vi "InitializeAnalogOutput.vi"(1 "AOTF":u16(ring) items=["None", "Laser 1", "Laser 2", "Laser 1 + 2", "Laser 3", "Laser 1 + 3", "Laser 2 + 3", "Laser 1+2+3", "Laser 1+2+3+4", "Laser 2+3+4"], 2 "% puls-duration":dbl=95.0, 3 "Image Settings":T1={"Start Position (µm)"={"x"=0.0, "y"=0.0, "z"=0.0}, "End Position (µm)"={"x"=10.0, "y"=10.0, "z"=0.0}, "Image Resolution (nm/pixel)"={"x"=50.0, "y"=50.0, "z"=100.0}, "Image Size (µm)"={"x"=10.0, "y"=10.0, "z"=0.0}, "Image Size (pixel)"={"x"=50, "y"=50, "z"=0}, "Time Resolution\n(ms/pixel)"=7.0, "1st Axis"=0, "2nd Axis"=1, "Retrace"=FALSE, "Estimated Time"=""} {"2nd Axis" items=["x", "y", "z"]; "1st Axis" items=["x", "y", "z"]; "Time Resolution\n(ms/pixel)" format="%.2f"; "Image Resolution (nm/pixel)"."z" format="%.2f"; "Image Resolution (nm/pixel)"."y" format="%.2f"; "Image Resolution (nm/pixel)"."x" format="%.2f"; "Image Size (µm)"."z" format="%.2f"; "Image Size (µm)"."y" format="%.2f"; "Image Size (µm)"."x" format="%.2f"; "End Position (µm)"."z" format="%.2f"; "End Position (µm)"."y" format="%.2f"; "End Position (µm)"."x" format="%.2f"; "Start Position (µm)"."z" format="%.2f"; "Start Position (µm)"."y" format="%.2f"; "Start Position (µm)"."x" format="%.2f"}, 4 "EOM":u16(ring) items=["None", "Trace", "Retrace", "All"]) -> (0 "Error out":errorcluster)   [LabVIEW 2009]
uses:
  ImageSettings.ctt
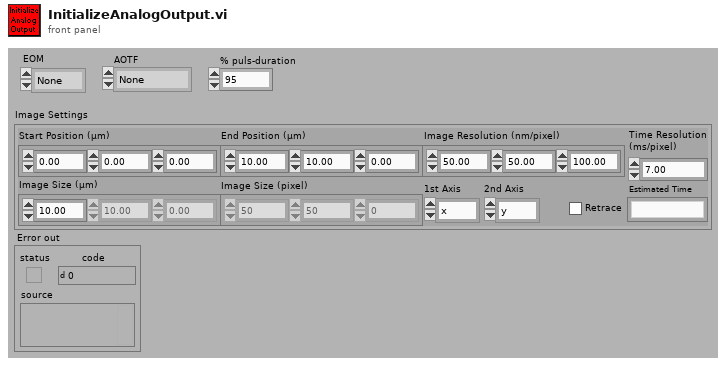
[diagram p1: front panel]
types:
  T1 = typedef "ImageSettings.ctt" = cluster{"Start Position (µm)":cluster{"x":dbl, "y":dbl, "z":dbl}, "End Position (µm)":cluster{"x":dbl, "y":dbl, "z":dbl}, "Image Resolution (nm/pixel)":cluster{"x":dbl, "y":dbl, "z":dbl}, "Image Size (µm)":cluster{"x":dbl, "y":dbl, "z":dbl}, "Image Size (pixel)":cluster{"x":u32, "y":u32, "z":u32}, "Time Resolution\n(ms/pixel)":dbl, "1st Axis":u16, "2nd Axis":u16, "Retrace":bool, "Estimated Time":string}
  T2 = typedef "AnalogSettings.ctt" = cluster{"PCI 671x Device Number":u32, "Samples per Unit":u32}
  T3 = typedef "AnalogTrace.ctt" = cluster{"Used":bool, "Waveform":waveform(dbl)}
  T4 = cluster{"new plane step[0]":dbl, "new plane step[1]":dbl, "new plane step[2]":dbl}
  T5 = typedef "LineScanStatus.ctt" = cluster{"in line":bool, "line status":cluster{"count":u32, "current":cluster{"x":u32, "y":u32, "z":u32}}, "plane status":cluster{"count":u32, "current":cluster{"x":u32, "y":u32, "z":u32}}, "new line step":cluster{"x":dbl, "y":dbl, "z":dbl}, "new plane step":cluster{"x":dbl, "y":dbl, "z":dbl}}
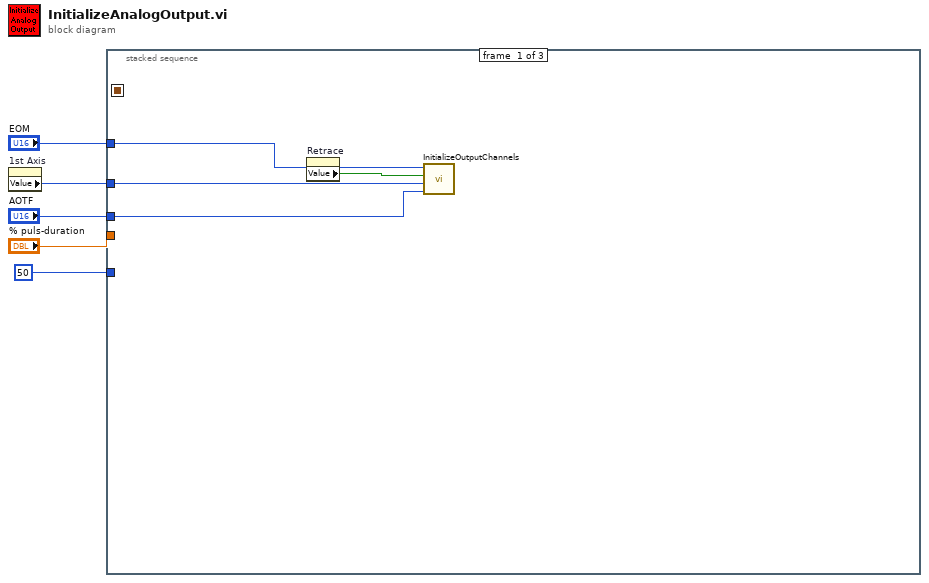
[diagram p0: block diagram]
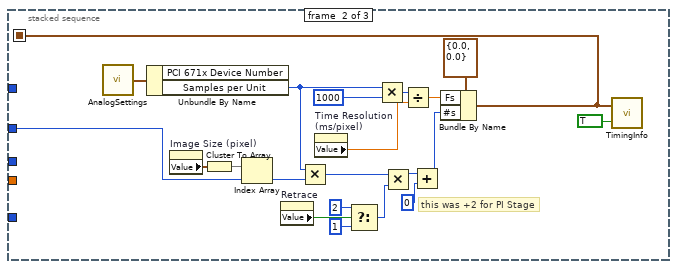
[diagram p2: hidden frame]
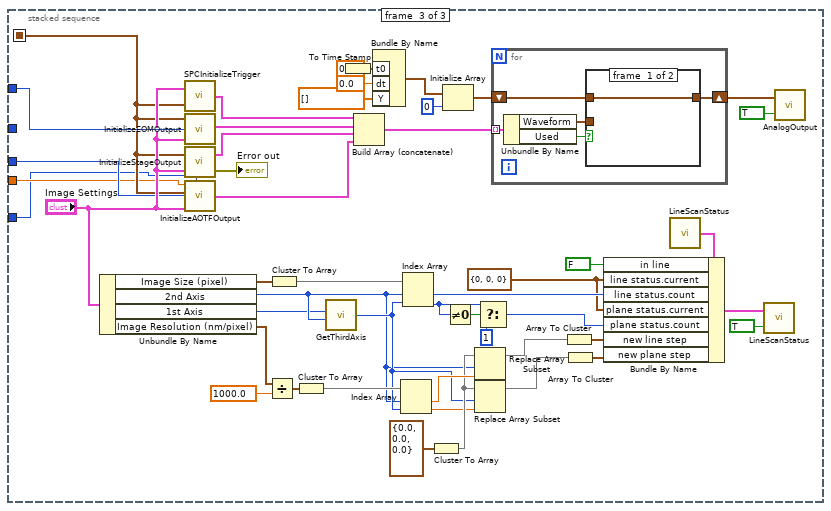
[diagram p3: hidden frame]
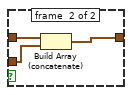
[diagram p4: hidden frame]
diagram:
  n1 = property on="1st Axis" class="Ring (strict)"() -> ("Value"=w5:u16)  [unwired: 2 in, 2 out]
  n2 = stacked-sequence {
    seq-local: [_ w10 _] -> [_ _ w36]
    tunnel: w5 -> [w9 w20 _]
    tunnel: "EOM" -> [w8 _ w74]
    tunnel: "AOTF" -> [w6 _ w35]
    tunnel: "% puls-duration" -> [_ _ w32]
    tunnel: u8 50 ("% rel. duration") -> [_ _ w31]
    frame #0 {
      n3 = property on="Retrace" class="Boolean (strict)"() -> ("Value"=w7:bool)  [unwired: 2 in, 2 out]
      n4 = call "InitializeOutputChannels.vi"("AOTF"=w6, "1st Axis"=w9, "Retrace"=w7, "EOM"=w8) -> ()
    }
    frame #1 {
      # "this was +2 for PI Stage"
      n5 = call "AnalogSettings.vi"() -> ("Analog Settings (output)"=w30:T2)  [unwired: 2 in]
      n6 = Unbundle By Name(w30) -> ("Samples per Unit"=w27:u32)  [unwired: 1 out]
      n7 = property on="Image Size (pixel)" class="Cluster (strict)"() -> ("Value"=w22:cluster{"x":u32, "y":u32, "z":u32})  [unwired: 2 in, 2 out]
      n8 = Cluster To Array(cluster=w22) -> (array=w21:u32[])
      n9 = Index Array(array=w21, index=w20) -> (element=w19:u32)
      n10 = property on="Retrace" class="Boolean (strict)"() -> ("Value"=w16:bool)  [unwired: 2 in, 2 out]
      n11 = Multiply(x=w27, y=w19) -> (x*y=w18:u32)
      n12 = property on="Time Resolution\n(ms/pixel)" class="Digital (strict)"() -> ("Value"=w23:dbl)  [unwired: 2 in, 2 out]
      n13 = Select(t=u32 2 ("x"), s=w16, f=u32 1 ("x")) -> (s? t:f=w17:u32)
      n14 = Multiply(x=w27, y=u32 1000 ("x")) -> (x*y=w28:u32)
      n15 = Multiply(x=w18, y=w17) -> (x*y=w12:u32)
      n16 = Divide(x=w28, y=w23) -> (x/y=w26:dbl)
      n17 = Add(x=w12, y=u32 0) -> (x+y=w13:u32)
      n18 = Bundle By Name(cluster=cluster{"Fs":dbl, "#s":dbl} {"Fs"=0.0, "#s"=0.0} ("Timing Info"), "Fs"=w26, "#s"=w13) -> (w10:cluster{"Fs":dbl, "#s":dbl})
      n19 = call "TimingInfo.vi"("Get/Set"=TRUE, "Timing Info (input)"=w10) -> ()  [unwired: 1 out]
    }
    frame #2 {
      w67 = cluster{"x":u32, "y":u32, "z":u32} {"x"=0, "y"=0, "z"=0} ("line status.current")
      n20 = Unbundle By Name("Image Settings") -> ("Image Size (pixel)"=w70:cluster{"x":u32, "y":u32, "z":u32}, "2nd Axis"=w51:u16, "1st Axis"=w50:u16, "Image Resolution (nm/pixel)"=w64:cluster{"x":dbl, "y":dbl, "z":dbl})
      n21 = call "SPCInitializeTrigger.vi"("timing info"=w36, "Image Settings"="Image Settings") -> ("signal out"=w76:T3)
      n22 = call "InitializeEOMOutput.vi"("Image Settings"="Image Settings", "EOM"=w74, "Timing Info"=w36) -> ("Analog Output"=w78:T3)
      n23 = call "InitializeStageOutput.vi"("Image Settings"="Image Settings", "Timing Info"=w36) -> ("Error out"=→"Error out":errorcluster, "Analog Output"=w77:T3)
      n24 = call "InitializeAOTFOutput.vi"("% puls-duration"=w32, "Timing Info"=w36, "AOTF"=w35, "Image Settings"="Image Settings", "% rel. duration"=w31) -> ("Array"=w34:T3[])
      n25 = Divide(x=w64, y=1000.0 ("t")) -> (x/y=w63:cluster{"x":dbl, "y":dbl, "z":dbl})
      n26 = Cluster To Array(cluster=w70) -> (array=w69:u32[])
      n27 = Cluster To Array(cluster=w63) -> (array=w62:dbl[])
      n28 = call "GetThirdAxis.vi"("1st Axis"=w51, "2nd Axis"=w50) -> ("3rd Axis"=w53:i32)  [unwired: 2 in]
      n29 = To Time Stamp(1:0.0 ("t0")) -> (0:w33:timestamp)
      n30 = Build Array (concatenate)(w76, w78, w77, w34) -> (w52:T3[])
      n31 = Bundle By Name("t0"=w33, "dt"=0.0, "Y"=dbl[] []) -> (w48:waveform(dbl))  [unwired: 1 in]
      n32 = Index Array(array=w62, index #1=w51, index #2=w53) -> (element #1=w60:dbl, element #2=w56:dbl)
      n33 = Index Array(array=w69, index #1=w51, index #2=w53) -> (element #1=w68:u32, element #2=w42:u32)
      n34 = Cluster To Array(cluster=cluster{"x":dbl, "y":dbl, "z":dbl} {"x"=0.0, "y"=0.0, "z"=0.0} ("new plane step")) -> (array=w57:dbl[])
      n35 = Initialize Array(w48, 0 ("dimension size")) -> (w49:waveform(dbl)[])
      n36 = Not Equal To 0?(x=w42) -> (x != 0?=w43:bool)
      n37 = Replace Array Subset(array=w57, new element=w60, index=w51) -> (w58:dbl[])
      n38 = Replace Array Subset(array=w57, new element=w56, index=w53) -> (w54:dbl[])
      n39 = Select(t=w42, s=w43, f=u32 1) -> (s? t:f=w40:u32)
      n40 = for {
        shift-right: [w81] -> w38
        shift-left: w49 -> [w80]
        tunnel: w52 -> [w83] mode=indexing
        n41 = Unbundle By Name(w83) -> ("Waveform"=w79:waveform(dbl), "Used"=w82:bool)
        n42 = case shown="True" w82 {
          tunnel: [w84 w87] -> w81
          tunnel: w80 -> [w84 w86]
          tunnel: w79 -> [_ w85]
          frame #0 {
          }
          frame #1 {
            n43 = Build Array (concatenate)(w86, w85) -> (w87:waveform(dbl)[])
          }
        }
      }
      n44 = Array To Cluster(array=w58) -> (cluster=w59:T4)
      n45 = Array To Cluster(array=w54) -> (cluster=w55:T4)
      n46 = call "LineScanStatus.vi"() -> ("Linescan Status (output)"=w66:T5)  [unwired: 2 in]
      n47 = Bundle By Name(cluster=w66, "in line"=FALSE, "line status.current"=w67, "line status.count"=w68, "plane status.current"=w67, "plane status.count"=w40, "new line step"=w59, "new plane step"=w55) -> (w72:T5)
      n48 = call "LineScanStatus.vi"("Get/Set"=TRUE, "Linescan Status (input)"=w72) -> ()  [unwired: 1 out]
      n49 = call "AnalogOutput.vi"("Get/Set"=TRUE, "Analog Output (input)"=w38) -> ()  [unwired: 1 out]
    }
  }
